vi "draw.vi"(0 "reference in":refnum<class "VINode.lvclass">, 1 "graphics":refnum<class "Graphics.lvclass">, 5 "error in (no error)":errorcluster) -> (14 "reference out":refnum<class "VINode.lvclass">, 19 "error out":errorcluster)   [LabVIEW 2014, in "VINode.lvclass"]
doc: "public void draw(Graphics2D g2, Point2D p, Point2D q)"
uses:
  <resource>/Framework/Providers/Open_GDS/UML/VINode_class/VINode.lvclass
  <resource>/Framework/Providers/Open_GDS/UML/Graphics_class/Graphics.lvclass
  <resource>/Framework/Providers/Open_GDS/UML/General/Rectangle/Rectangle Rectangle2D.ctl
  <resource>/Framework/Providers/Open_GDS/UML/UMLEditor/UMLEditor_StoredColors.ctl
  <resource>/Framework/Providers/Open_GDS/UML/MultiLineString_class/MultiLineString.lvclass
  <resource>/Framework/Providers/Open_GDS/UML/RectangularNode_class/RectangularNode.lvclass
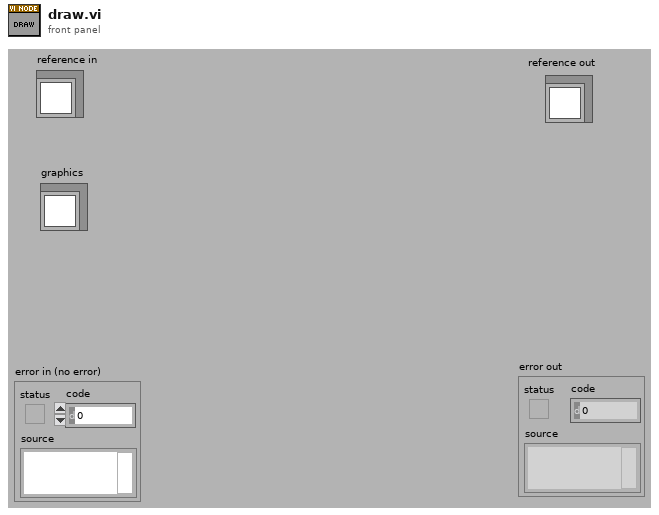
[diagram p1: front panel]
types:
  T1 = typedef "UMLEditor_StoredColors.ctl" = enum16{"ClassBackgroudColor", "ClassBackgroudColorWithClassPath", "ClassBackgroudColorForApplicationVIStereotype", "ClassBackgroudColorForTypeStereotype", "StateBackgroudColor"}
  T2 = typedef "Rectangle Rectangle2D.ctl" = cluster{"x":dbl, "y":dbl, "width":dbl, "height":dbl}
  T3 = typedef "VINode.lvclass/ObjectAttributes.ctl" = cluster{"midHeight":dbl, "botHeight":dbl, "Name":refnum<class "MultiLineString.lvclass">, "DEFAULT_COMPARTMENT_HEIGHT":i32, "DEFAULT_WIDTH":i32, "DEFAULT_HEIGHT":i32, "ClassPath":path, "Icon":u8[][], "Description":refnum<class "MultiLineString.lvclass">, "ShowDescription":bool}
  T4 = typedef "RectangularNode.lvclass/ObjectAttributes.ctl" = cluster{"bounds":T2}
  T5 = typedef "Point Point2D.ctl" = cluster{"x":dbl, "y":dbl}
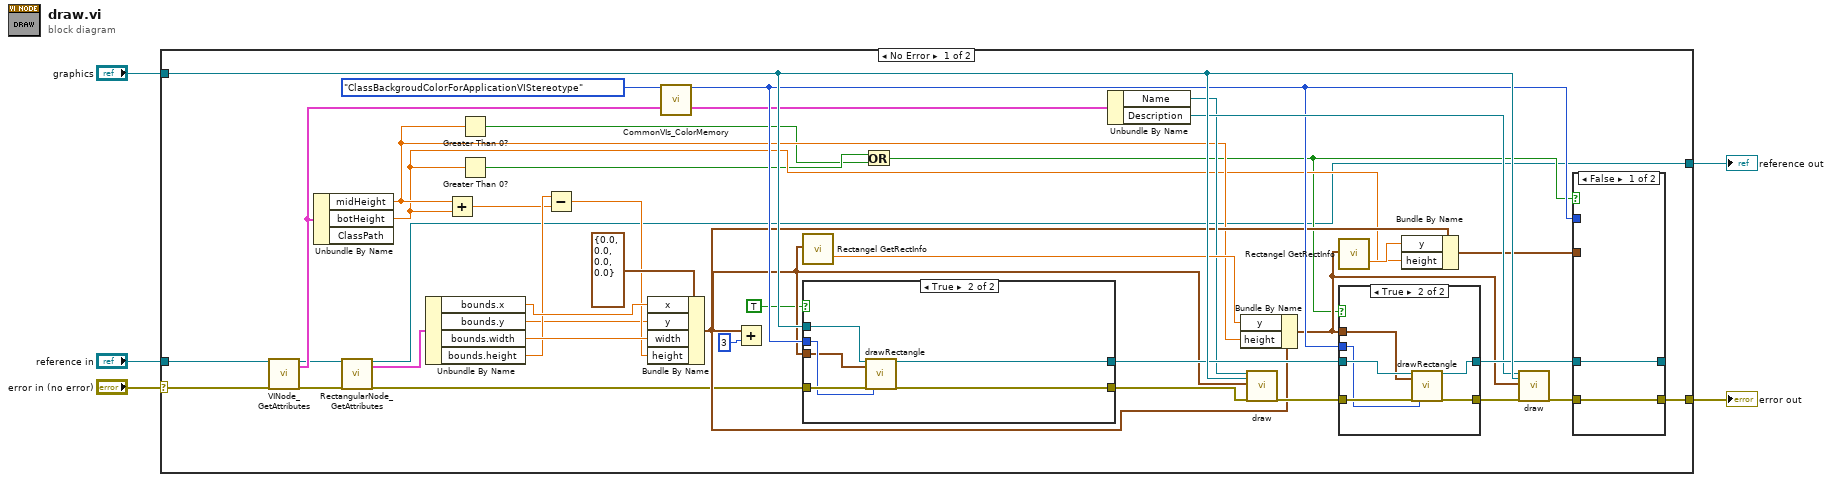
[diagram p0: block diagram]
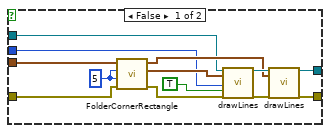
[diagram p2: hidden frame]
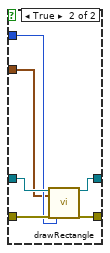
[diagram p3: hidden frame]
diagram:
  n1 = case shown="No Error" "error in (no error)" {
    selector: "error in (no error)" -> [w42 w80]
    tunnel: "reference in" -> [w44 w81]
    tunnel: [w6 w80] -> w4
    tunnel: [w9 w81] -> w3
    tunnel: "graphics" -> [w43 _]
    frame No Error {
      n2 = call <resource>:"VINode_GetAttributes.vi"("reference in"=w44, "error in (no error)"=w42) -> ("reference out"=w11:refnum<class "VINode.lvclass">, "Data"=w12:T3, "error out"=w10:errorcluster)  [unwired: 1 in, 14 out]
      n3 = Unbundle By Name(w12) -> ("midHeight"=w18:dbl, "botHeight"=w17:dbl)  [unwired: 1 out]
      n4 = call <resource>:"RectangularNode_GetAttributes.vi"("reference in"=w11, "error in (no error)"=w10) -> ("reference out"=w9:refnum<class "VINode.lvclass">, "Data"=w8:T4, "error out"=w7:errorcluster)  [unwired: 14 in, 1 out]
      n5 = Unbundle By Name(w8) -> ("bounds.x"=w40:dbl, "bounds.y"=w36:dbl, "bounds.width"=w39:dbl, "bounds.height"=w38:dbl)
      n6 = Add(x=w18, y=w17) -> (x+y=w35:dbl)
      n7 = Greater Than 0?(x=w18) -> (x > 0?=w14:bool)
      n8 = Greater Than 0?(x=w17) -> (x > 0?=w15:bool)
      n9 = Subtract(x=w38, y=w35) -> (x-y=w37:dbl)
      n10 = Bundle By Name(cluster=T2 {"x"=0.0, "y"=0.0, "width"=0.0, "height"=0.0} ("points"), "x"=w40, "y"=w36, "width"=w39, "height"=w37) -> (w20:T2)
      n11 = call <resource>:"CommonVIs_ColorMemory.vi"("ColorName"=UMLEditor_StoredColors."ClassBackgroudColorForApplicationVIStereotype" ("UMLPathes")) -> ("Color Out"=w24:u32)  [unwired: 3 in, 15 out]
      n12 = Add(x=w20, y=3) -> ()  [unwired: 1 out]
      n13 = call <resource>:"Rectangel GetRectInfo.vi"("bounds"=w20) -> ("maxY"=w27:dbl)  [unwired: 1 in, 17 out]
      n14 = case shown="True" TRUE {
        tunnel: w43 -> [w51 w63]
        tunnel: [w50 w62] -> w34
        tunnel: [w49 w61] -> w32
        tunnel: w7 -> [w45 w60]
        tunnel: w24 -> [w48 w59]
        tunnel: w20 -> [w47 w58]
        frame False {
          w46 = 5 ("FOLD_X")
          n15 = call <resource>:"FolderCornerRectangle.vi"("error out 2"=w45, "FOLD_Y"=w46, "FOLD_X"=w46, "bounds"=w47) -> ("error out"=w53:errorcluster, "Array 2"=w57:T5[], "Array"=w54:T5[])  [unwired: 5 out]
          n16 = call <resource>:"drawLines.vi"("reference"=w51, "points"=w57, "color(if not used=default color)"=w48, "fill?(F)"=TRUE, "error in (no error)"=w53) -> ("reference out"=w56:refnum<class "Graphics.lvclass">, "error out"=w55:errorcluster)  [unwired: 2 in, 11 out]
          n17 = call <resource>:"drawLines.vi"("reference"=w56, "points"=w54, "error in (no error)"=w55) -> ("reference out"=w50:refnum<class "Graphics.lvclass">, "error out"=w49:errorcluster)  [unwired: 4 in, 11 out]
        }
        frame True {
          n18 = call <resource>:"drawRectangle.vi"("reference"=w63, "rectangle"=w58, "error in (no error)"=w60, "FillClor(if not used=BorderColorIsUsed,AutoFill)"=w59) -> ("reference out"=w62:refnum<class "Graphics.lvclass">, "error out"=w61:errorcluster)  [unwired: 3 in, 11 out]
        }
      }
      n19 = Or(x=w15, y=w14) -> (x .or. y?=w13:bool)
      n20 = Unbundle By Name(w12) -> ("Name"=w25:refnum<class "MultiLineString.lvclass">, "Description"=w28:refnum<class "MultiLineString.lvclass">)
      n21 = Bundle By Name(cluster=w20, "y"=w27, "height"=w18) -> (w19:T2)
      n22 = call-dynamic "draw.vi"("reference"=w25, "graphics"=w43, "bounds"=w20, "error in (no error)"=w32) -> ("error out"=w31:errorcluster)  [unwired: 14 in, 1 out]
      n23 = call <resource>:"Rectangel GetRectInfo.vi"("bounds"=w19) -> ("maxY"=w26:dbl)  [unwired: 1 in, 17 out]
      n24 = case shown="True" w13 {
        tunnel: w34 -> [w73 w79]
        tunnel: [w73 w78] -> w33
        tunnel: w31 -> [w72 w77]
        tunnel: [w72 w76] -> w30
        tunnel: w24 -> [_ w75]
        tunnel: w19 -> [_ w74]
        frame False {
        }
        frame True {
          n25 = call <resource>:"drawRectangle.vi"("reference"=w79, "rectangle"=w74, "error in (no error)"=w77, "FillClor(if not used=BorderColorIsUsed,AutoFill)"=w75) -> ("reference out"=w78:refnum<class "Graphics.lvclass">, "error out"=w76:errorcluster)  [unwired: 3 in, 11 out]
        }
      }
      n26 = Bundle By Name(cluster=w20, "y"=w26, "height"=w17) -> (w22:T2)
      n27 = call-dynamic "draw.vi"("reference"=w28, "graphics"=w43, "bounds"=w19, "error in (no error)"=w30) -> ("error out"=w29:errorcluster)  [unwired: 14 in, 1 out]
      n28 = case shown="False" w13 {
        tunnel: w33 -> [w64 w71]
        tunnel: w29 -> [w65 w70]
        tunnel: [w65 w69] -> w6
        tunnel: w24 -> [_ w68]
        tunnel: w22 -> [_ w67]
        tunnel: [w64 w66] -> _
        frame False {
        }
        frame True {
          n29 = call <resource>:"drawRectangle.vi"("reference"=w71, "rectangle"=w67, "error in (no error)"=w70, "FillClor(if not used=BorderColorIsUsed,AutoFill)"=w68) -> ("reference out"=w66:refnum<class "Graphics.lvclass">, "error out"=w69:errorcluster)  [unwired: 3 in, 11 out]
        }
      }
    }
    frame Error {
    }
  }
  "reference out" <- w3
  "error out" <- w4
